vi "UtrasonicCorrection.vi"(7 "Y_dis(mm)":dbl=100.0, 8 "Error In":errorcluster) -> (0 "Error Out":errorcluster)   [LabVIEW 2019]
uses:
  <vilib>/Platform/TimedLoop/XDataNode/timing_clust.ctl
  <vilib>/Platform/TimedLoop/XDataNode/nitl_modes.ctl
  <vilib>/Platform/TimedLoop/XDataNode/wakeup.ctl
  <vilib>/addons/control/pid/pid.llb/PID (DBL).vi
  <vilib>/platform/TimedLoop/XDataNode/XDataNode.xnode
  WSCbot_V3_Toolkit.lvlibp
  <vilib>/addons/control/pid/NI_PID_pid.lvlib
  <vilib>/Platform/TimedLoop/XDataNode/XDNodeRunTimeDep.lvlib
panel:
  in  "Error":dbl=-0.055
  out "Distance_L(mm)":dbl=97.19533125
  out "Distance_R(mm)":dbl=91.92083625
  in  "Stop Button":bool
  out "Boolean 2":bool=TRUE
  out "Boolean":bool=TRUE
  in  "PID 前後":T1={"proportional gain (Kc)"=1.5, "integral time (Ti, min)"=0.0, "derivative time (Td, min)"=0.0001} {"derivative time (Td, min)" format="%#.6f"; "integral time (Ti, min)" format="%#.3f"; "proportional gain (Kc)" format="%#.3f"}
  in  "PID 自旋":T1={"proportional gain (Kc)"=1.5, "integral time (Ti, min)"=0.0, "derivative time (Td, min)"=1e-05} {"derivative time (Td, min)" format="%#.6f"; "integral time (Ti, min)" format="%#.3f"; "proportional gain (Kc)" format="%#.3f"}
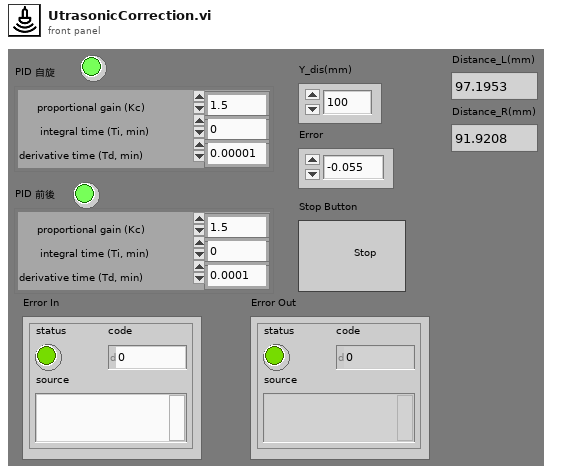
[diagram p1: front panel]
types:
  T1 = cluster{"proportional gain (Kc)":dbl, "integral time (Ti, min)":dbl, "derivative time (Td, min)":dbl}
  T2 = typedef "XDNodeRunTimeDep.lvlib/timing_clust.ctl" = cluster{"Expected End [f-1]":u64, "Actual End [f-1]":u64, "Finished Late? [f-1]":bool, "Expected End [i-1]":u64, "Actual End [i-1]":u64, "Finished Late? [i-1]":bool, "Expected Start [i]":u64, "Actual Start [i]":u64, "Expected Start [f]":u64, "Actual Start [f]":u64, "Source Name":string, "Structure Name":string, "Period":i64, "Deadline":i64, "Offset":i64, "Start":i64, "Priority":i32, "Timeout":i32, "Mode":T3, "Wakeup Reason":T4, "Error":errorcluster, "Source Type":string, "Secondary Source Type":string, "Global End Time":u64, "Global Start Time":u64, "Frame Duration":u64, "Iteration Duration":u64, "Assigned CPU":i32, "I/O Scan Engine Mode":u32}
  T3 = typedef "XDNodeRunTimeDep.lvlib/nitl_modes.ctl" = enum32{"No Change", "Process missed periods, maintain original phase", "Discard missed periods, maintain original phase", "Process missed periods, ignore original phase", "Discard missed periods, ignore original phase"}
  T4 = typedef "XDNodeRunTimeDep.lvlib/wakeup.ctl" = enum32{"Normal", "Aborted", "Asynchronous wakeup", "Timing source error", "Timed loop error", "Timeout"}
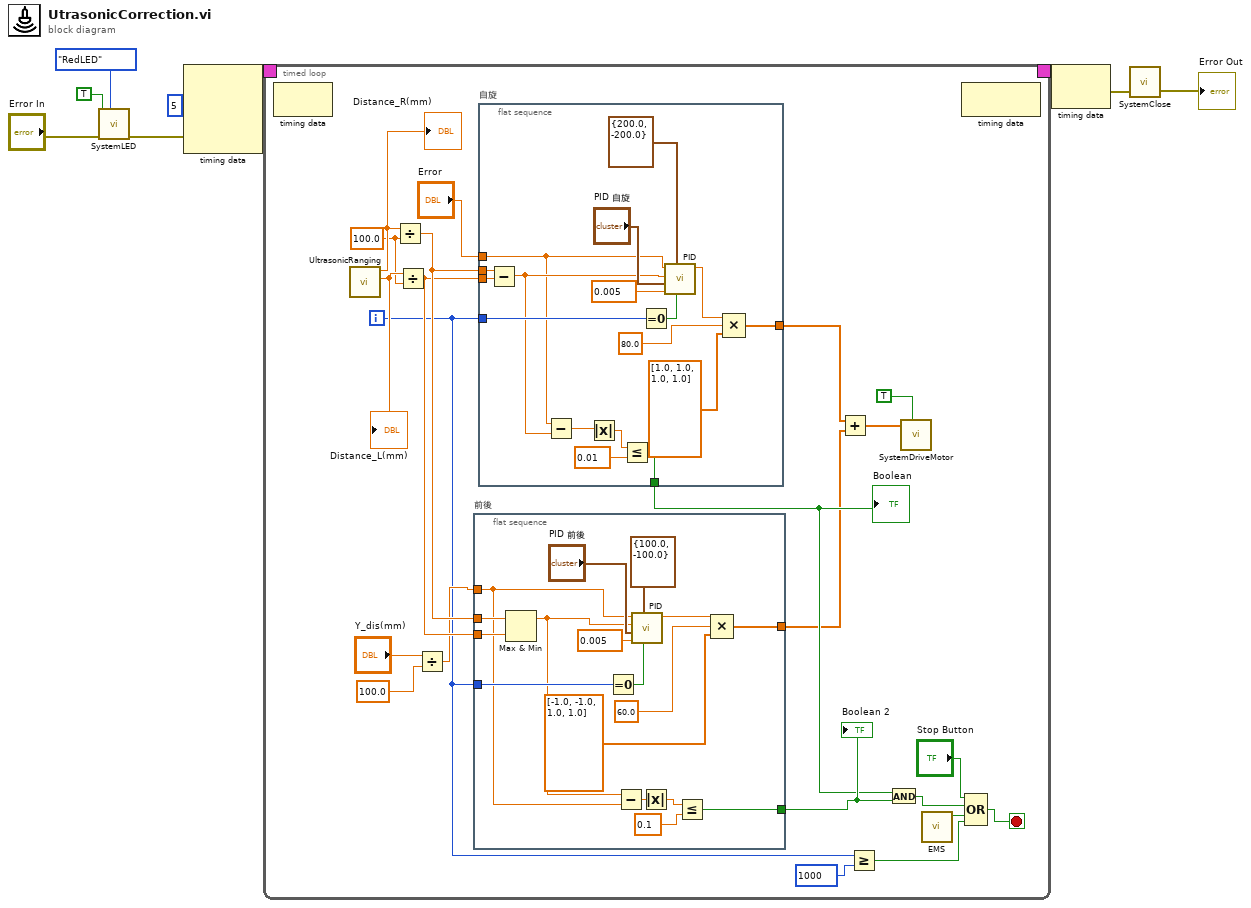
[diagram p0: block diagram]
diagram:
  n1 = call "SystemLED.vi"("SelectColor"=enum16{"RedLED", "GreenLED", "YellowLED"}."RedLED", "error in"="Error In", "Set"=TRUE) -> ("error out"=w6:errorcluster)  [unwired: 8 in]
  n2 = node-c288(i64 5 ("Period"), w6) -> (w9:T2)  [unwired: 2 in]
  n3 = timed-loop {
    timing: w9 -> [_]
    timing-out: [_] -> w8
    i -> [w12]
    stop <- w27 stop-if-true
    w18 = 100.0 ("y")
    n4 = node-c288() -> ()  [unwired: 1 in, 1 out]
    n5 = call "UltrasonicRanging.vi"() -> ("Distance_L(mm)"=w20:dbl, "Distance_R(mm)"=w22:dbl)  [unwired: 9 in, 1 out]
    "Distance_R(mm)" <- w22
    "Distance_L(mm)" <- w20
    n6 = Divide(x=w22, y=w18) -> (x/y=w21:dbl)
    n7 = Divide(x=w20, y=w18) -> (x/y=w19:dbl)
    n8 = Divide(x="Y_dis(mm)", y=100.0) -> (x/y=w15:dbl)
    n9 = flat-sequence "前後" {
      tunnel: w21 -> [w48]
      tunnel: w19 -> [w47]
      tunnel: w15 -> [w37]
      tunnel: w12 -> [w44]
      tunnel: [w35] -> w31
      tunnel: [w34] -> w28
      frame #0 {
        n10 = Max & Min(x=w48, y=w47) -> (max(x,y)=w38:dbl)  [unwired: 1 out]
        n11 = Equal To 0?(x=w44) -> (x = 0?=w43:bool)
        n12 = Subtract(x=w38, y=w37) -> (x-y=w33:dbl)
        n13 = call-poly <vilib>:"PID.vi"("reinitialize? (F)"=w43, "output range"=cluster{"output high":dbl, "output low":dbl} {"output high"=100.0, "output low"=-100.0}, "dt (s)"=0.005, "PID gains"="PID 前後", "process variable"=w38, "setpoint"=w37) -> ("output"=w41:dbl)  [unwired: 4 in, 1 out]
        n14 = Absolute Value(x=w33) -> (abs(x)=w32:dbl)
        n15 = Less Or Equal?(x=w32, y=0.1) -> (x <= y?=w35:bool)
        n16 = Compound Arithmetic op=MULTIPLY(w41, 60.0 ("dt (s)"), dbl[] [-1.0, -1.0, 1.0, 1.0]) -> (w34:dbl[])
      }
    }
    n17 = flat-sequence "自旋" {
      tunnel: w12 -> [w62]
      tunnel: w21 -> [w57]
      tunnel: w19 -> [w56]
      tunnel: [w54] -> w30
      tunnel: [w53] -> w29
      tunnel: "Error" -> [w49]
      frame #0 {
        n18 = Subtract(x=w57, y=w56) -> (x-y=w50:dbl)
        n19 = Subtract(x=w49, y=w50) -> (x-y=w51:dbl)
        n20 = Absolute Value(x=w51) -> (abs(x)=w52:dbl)
        n21 = Less Or Equal?(x=w52, y=0.01) -> (x <= y?=w54:bool)
        n22 = Equal To 0?(x=w62) -> (x = 0?=w61:bool)
        n23 = call-poly <vilib>:"PID.vi"("reinitialize? (F)"=w61, "output range"=cluster{"output high":dbl, "output low":dbl} {"output high"=200.0, "output low"=-200.0}, "dt (s)"=0.005, "PID gains"="PID 自旋", "process variable"=w50, "setpoint"=w49) -> ("output"=w60:dbl)  [unwired: 4 in, 1 out]
        n24 = Compound Arithmetic op=MULTIPLY(w60, 80.0 ("dt (s)"), dbl[] [1.0, 1.0, 1.0, 1.0]) -> (w53:dbl[])
      }
    }
    n25 = Add(x=w29, y=w28) -> (x+y=w24:dbl[])
    n26 = Greater Or Equal?(x=w12, y=1000) -> (x >= y?=w10:bool)
    n27 = And(x=w30, y=w31) -> (x .and. y?=w25:bool)
    n28 = call "SystemDriveMotor.vi"("Enable?"=TRUE, "4xMotor(deg/s)"=w24) -> ()  [unwired: 8 in, 2 out]
    n29 = call "EMS.vi"() -> ("EMS"=w26:bool)  [unwired: 10 in, 1 out]
    n30 = node-c288() -> ()  [unwired: 1 in, 1 out]
    n31 = Compound Arithmetic op=OR("Stop Button", w25, w26, w10) -> (w27:bool)
    "Boolean" <- w30
    "Boolean 2" <- w31
  }
  n32 = node-c288(w8) -> (w2:errorcluster)
  n33 = call "SystemClose.vi"("error in"=w2) -> ("error out"=→"Error Out":errorcluster)  [unwired: 2 in]
